vi "LED Sequence.vi"(9 "Tag Name":string="Boolean processing result 0", 10 "Name":string="Led Sequence") -> (2 "Sequence out":refnum<class "Sequence Config.lvclass">)   [LabVIEW 2015, in "Sequencer Module tests.lvlib"]
uses:
  Sequencer Module tests.lvlib
  classes/Sequence Config/Sequence Config.lvclass
  <vilib>/NI/Tag Bus/tag/Data Type.ctl
  classes/Wait Step Config/Wait Step Config.lvclass
  classes/Update Tag Step Config/Update Tag Configuration/Update Tag Config.lvclass
  <vilib>/NI/Tag Bus Module Framework/channel/channel classification.ctl
  <vilib>/NI/Tag Bus/tag/tag descriptor.lvclass
  <vilib>/NI/Tag Bus Module Framework/channel/TBM channel.lvclass
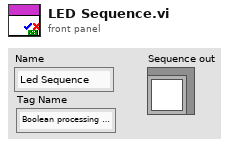
[diagram p1: front panel]
types:
  T1 = typedef "TBM channel.lvclass/channel classification.ctl" = enum16{"input data", "output data", "processing parameter", "processing result"}
  T2 = typedef "tag bus.lvlib/tag descriptor.lvclass/Data Type.ctl" = enum16{"Double", "Single", "I64", "I32", "I16", "I8", "U64", "U32", "U16", "U8", "Boolean", "String", "Array of Double", "Array of Single", "Array of I64", "Array of I32", "Array of I16", "Array of I8", "Array of U64", "Array of U32", "Array of U16", "Array of U8", "Array of Boolean", "Array of String"}
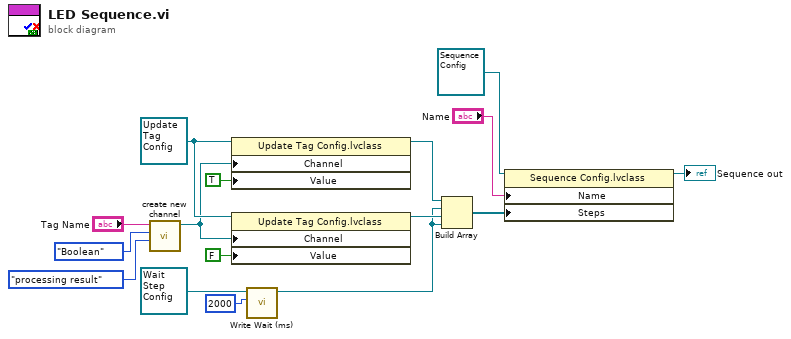
[diagram p0: block diagram]
diagram:
  w8 = refnum<class "Update Tag Config.lvclass"> refnum ("Update Tag Config.lvclass")
  n1 = call <vilib>:"create new channel.vi"("channel classification"=channel_classification."processing result", "data type"=Data_Type."Boolean" ("Data Type"), "channel name"="Tag Name") -> ("channel"=w4:refnum<class "TBM channel.lvclass">)  [unwired: 8 in]
  n2 = property class="Update Tag Config.lvclass"(reference=w8, "Channel"=w4, "Value"=TRUE) -> (reference out=w15:refnum<class "Update Tag Config.lvclass">)  [unwired: 1 in, 1 out]
  n3 = property class="Update Tag Config.lvclass"(reference=w8, "Channel"=w4, "Value"=FALSE) -> (reference out=w16:refnum<class "Update Tag Config.lvclass">)  [unwired: 1 in, 1 out]
  n4 = call-dynamic "Write Wait (ms).vi"("Wait (ms)"=u32 2000, "Wait Step in"=refnum<class "Wait Step Config.lvclass"> refnum ("Wait Step Config.lvclass")) -> ("Wait Step out"=w1:refnum<class "Wait Step Config.lvclass">)  [unwired: 8 in, 1 out]
  n5 = Build Array(w15, w1, w16, w1) -> (w14:refnum<class "Step Config.lvclass">[])
  n6 = property class="Sequence Config.lvclass"(reference=refnum<class "Sequence Config.lvclass"> refnum ("Sequence Config.lvclass"), "Name"="Name", "Steps"=w14) -> (reference out=→"Sequence out":refnum<class "Sequence Config.lvclass">)  [unwired: 1 in, 1 out]
